vi "Get ref name.vi"(9 "i":i32, 10 "step":i32, 11 "name":string) -> (3 "resources":string)   [LabVIEW 2010]
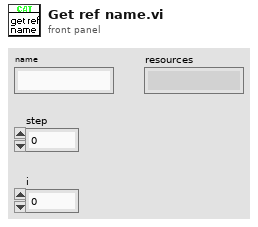
[diagram p1: front panel]
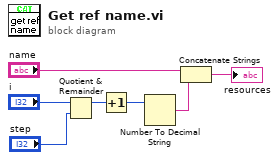
[diagram p0: block diagram]
diagram:
  n1 = Quotient & Remainder(x="i", y="step") -> (x-y*floor(x/y)=w4:i32)  [unwired: 1 out]
  n2 = Increment(x=w4) -> (x+1=w1:i32)
  n3 = Number To Decimal String(number=w1) -> (decimal integer string=w5:string)  [unwired: 1 in]
  n4 = Concatenate Strings("name", w5) -> (→"resources":string)
